vi "Set Wavelength.vi"(7 "Ref Wavelength":refnum<vi>, 8 "error in":errorcluster, 9 "Head Channel":i16, 10 "Pulsar Handle":i16, 11 "OphirFastX (in)":refnum<k7>) -> (0 "error out":errorcluster, 3 "OphirFastX (out)":refnum<k7>)   [LabVIEW 2009]
panel:
  # "Guillaume Plateau - yguig2@yahoo.fr"
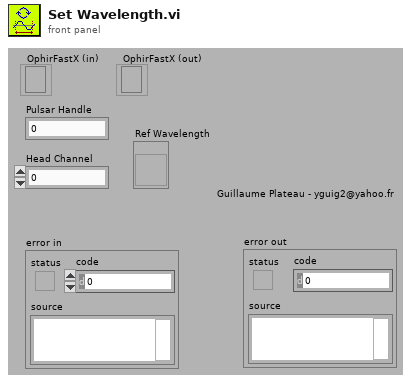
[diagram p1: front panel]
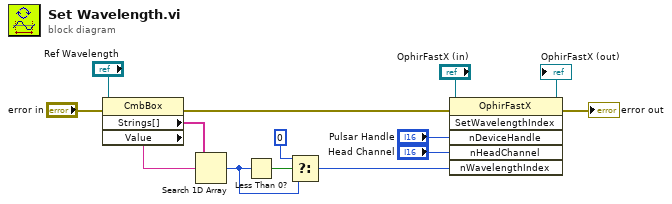
[diagram p0: block diagram]
diagram:
  n1 = property class="CmbBox"(reference="Ref Wavelength", error in="error in") -> (error out=w2:errorcluster, "Strings[]"=w6:string[], "Value"=w7:string)  [unwired: 1 out]
  n2 = Search 1D Array(1D array=w6, element=w7) -> (index of element=w10:i32)  [unwired: 1 in]
  n3 = Less Than 0?(x=w10) -> (x < 0?=w8:bool)
  n4 = Select(t=i16 0 ("nRangeIndex"), s=w8, f=w10) -> (s? t:f=w3:i32)
  n5 = invoke class="OphirFastX" method="SetWavelengthIndex"(reference="OphirFastX (in)", error in=w2, "nDeviceHandle"="Pulsar Handle", "nHeadChannel"="Head Channel", "nWavelengthIndex"=w3) -> (reference out=→"OphirFastX (out)":refnum<k7>, error out=→"error out":errorcluster)  [unwired: 1 in, 4 out]
